vi "CursorsRefresh.vi"(2 "Cursors簇句柄引用":refnum<vi>, 3 "Cursor字符串句柄引用":refnum<vi>) -> ()   [LabVIEW 2012]
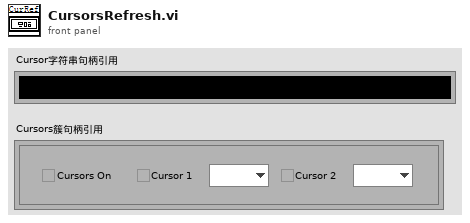
[diagram p1: front panel]
types:
  T1 = enum8{"Enabled", "Disabled", "Disabled and Grayed Out"}
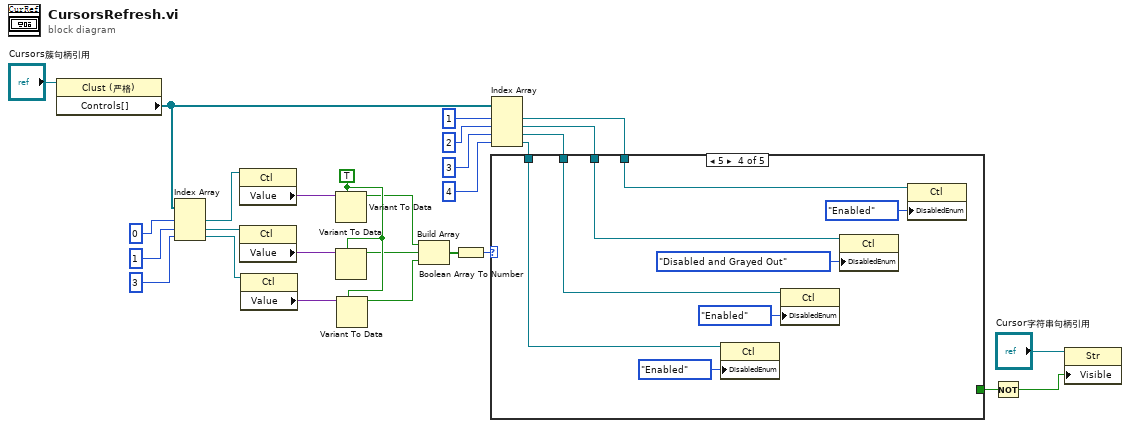
[diagram p0: block diagram]
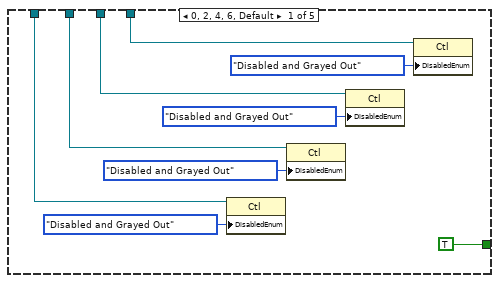
[diagram p2: hidden frame]
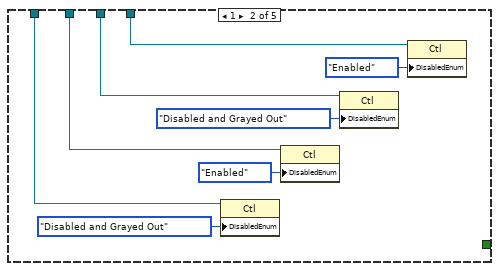
[diagram p3: hidden frame]
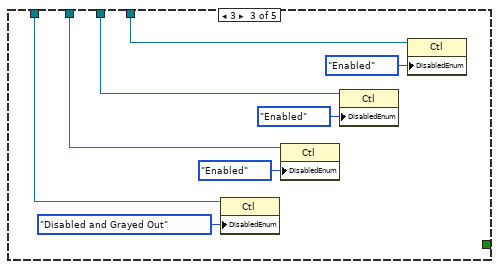
[diagram p4: hidden frame]
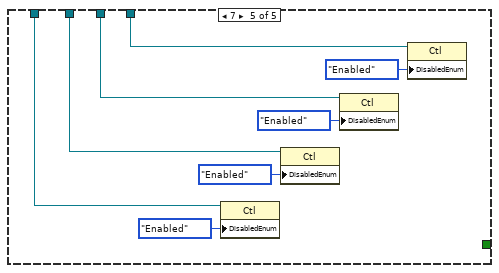
[diagram p5: hidden frame]
diagram:
  w18 = TRUE
  n1 = property class="Clust (严格)"(reference="Cursors簇句柄引用") -> ("Controls[]"=w4:refnum<vi>[])  [unwired: 1 in, 2 out]
  n2 = Index Array(array=w4, index #1=0 ("索引"), index #2=1 ("索引"), index #3=3) -> (element #1=w24:refnum<vi>, element #2=w23:refnum<vi>, element #3=w22:refnum<vi>)
  n3 = property class="Ctl"(reference=w24) -> ("Value"=w21:variant)  [unwired: 1 in, 2 out]
  n4 = property class="Ctl"(reference=w23) -> ("Value"=w20:variant)  [unwired: 1 in, 2 out]
  n5 = property class="Ctl"(reference=w22) -> ("Value"=w19:variant)  [unwired: 1 in, 2 out]
  n6 = Variant To Data(type=w18, Variant=w21) -> (data=w17:bool)  [unwired: 1 in, 1 out]
  n7 = Variant To Data(type=w18, Variant=w20) -> (data=w16:bool)  [unwired: 1 in, 1 out]
  n8 = Variant To Data(type=w18, Variant=w19) -> (data=w15:bool)  [unwired: 1 in, 1 out]
  n9 = Build Array(w17, w16, w15) -> (w14:bool[])
  n10 = Boolean Array To Number(Boolean array=w14) -> (number=w13:u32)
  n11 = Index Array(array=w4, index #1=1 ("索引"), index #2=2, index #3=3, index #4=4) -> (element #1=w8:refnum<vi>, element #2=w7:refnum<vi>, element #3=w6:refnum<vi>, element #4=w5:refnum<vi>)
  n12 = case shown="5" w13 {
    tunnel: w8 -> [w36 w41 w49 w54 w62]
    tunnel: w7 -> [w30 w40 w48 w55 w63]
    tunnel: w6 -> [w31 w39 w47 w56 w64]
    tunnel: w5 -> [w32 w38 w46 w57 w65]
    tunnel: [TRUE ("可见") _ _ _ _] -> w2
    frame 0, 2, 4, 6, Default {
      n13 = property class="Ctl"(reference=w32, "DisabledEnum"=T1."Disabled and Grayed Out" ("禁用")) -> ()  [unwired: 1 in, 2 out]
      n14 = property class="Ctl"(reference=w31, "DisabledEnum"=T1."Disabled and Grayed Out" ("禁用")) -> ()  [unwired: 1 in, 2 out]
      n15 = property class="Ctl"(reference=w30, "DisabledEnum"=T1."Disabled and Grayed Out" ("禁用")) -> ()  [unwired: 1 in, 2 out]
      n16 = property class="Ctl"(reference=w36, "DisabledEnum"=T1."Disabled and Grayed Out" ("禁用")) -> ()  [unwired: 1 in, 2 out]
    }
    frame 1 {
      n17 = property class="Ctl"(reference=w38, "DisabledEnum"=T1."Disabled and Grayed Out" ("禁用")) -> ()  [unwired: 1 in, 2 out]
      n18 = property class="Ctl"(reference=w39, "DisabledEnum"=T1."Enabled" ("禁用")) -> ()  [unwired: 1 in, 2 out]
      n19 = property class="Ctl"(reference=w40, "DisabledEnum"=T1."Disabled and Grayed Out" ("禁用")) -> ()  [unwired: 1 in, 2 out]
      n20 = property class="Ctl"(reference=w41, "DisabledEnum"=T1."Enabled" ("禁用")) -> ()  [unwired: 1 in, 2 out]
    }
    frame 3 {
      n21 = property class="Ctl"(reference=w46, "DisabledEnum"=T1."Disabled and Grayed Out" ("禁用")) -> ()  [unwired: 1 in, 2 out]
      n22 = property class="Ctl"(reference=w47, "DisabledEnum"=T1."Enabled" ("禁用")) -> ()  [unwired: 1 in, 2 out]
      n23 = property class="Ctl"(reference=w48, "DisabledEnum"=T1."Enabled" ("禁用")) -> ()  [unwired: 1 in, 2 out]
      n24 = property class="Ctl"(reference=w49, "DisabledEnum"=T1."Enabled" ("禁用")) -> ()  [unwired: 1 in, 2 out]
    }
    frame 5 {
      n25 = property class="Ctl"(reference=w57, "DisabledEnum"=T1."Enabled" ("禁用")) -> ()  [unwired: 1 in, 2 out]
      n26 = property class="Ctl"(reference=w56, "DisabledEnum"=T1."Enabled" ("禁用")) -> ()  [unwired: 1 in, 2 out]
      n27 = property class="Ctl"(reference=w55, "DisabledEnum"=T1."Disabled and Grayed Out" ("禁用")) -> ()  [unwired: 1 in, 2 out]
      n28 = property class="Ctl"(reference=w54, "DisabledEnum"=T1."Enabled" ("禁用")) -> ()  [unwired: 1 in, 2 out]
    }
    frame 7 {
      n29 = property class="Ctl"(reference=w65, "DisabledEnum"=T1."Enabled" ("禁用")) -> ()  [unwired: 1 in, 2 out]
      n30 = property class="Ctl"(reference=w64, "DisabledEnum"=T1."Enabled" ("禁用")) -> ()  [unwired: 1 in, 2 out]
      n31 = property class="Ctl"(reference=w63, "DisabledEnum"=T1."Enabled" ("禁用")) -> ()  [unwired: 1 in, 2 out]
      n32 = property class="Ctl"(reference=w62, "DisabledEnum"=T1."Enabled" ("禁用")) -> ()  [unwired: 1 in, 2 out]
    }
  }
  n33 = Not(x=w2) -> (.not. x?=w1:bool)
  n34 = property class="Str"(reference="Cursor字符串句柄引用", "Visible"=w1) -> ()  [unwired: 1 in, 2 out]
